vi "On Drop.vi"(8 "error in (no error)":errorcluster, 10 "Actor in":refnum<class "Actor.lvclass">, 11 "Client Connection Handler Msg in":refnum<class "Client Connection Handler Msg.lvclass">) -> (0 "error out":errorcluster, 2 "Actor out":refnum<class "Actor.lvclass">, 3 "Client Connection Handler Msg out":refnum<class "Client Connection Handler Msg.lvclass">)   [LabVIEW 2021, in "Echo Broadcast With Server Manager.lvlib" / "Client Connection Handler Msg.lvclass"]
uses:
  Client Connection Handler Msg.lvclass
  <vilib>/ActorFramework/Actor/Actor.lvclass
  WS Client Subscriber/WS Client Subscriber.lvclass
  C:/Program Files/National Instruments/LabVIEW 2021/vi.lib/ActorFramework/Actor/Actor.lvclass
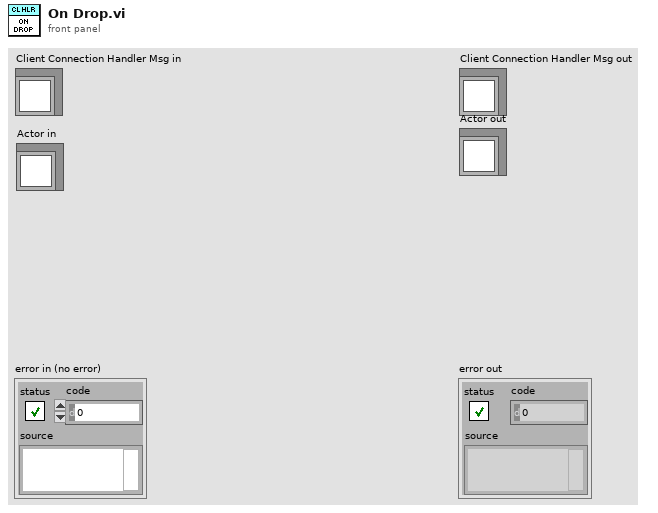
[diagram p1: front panel]
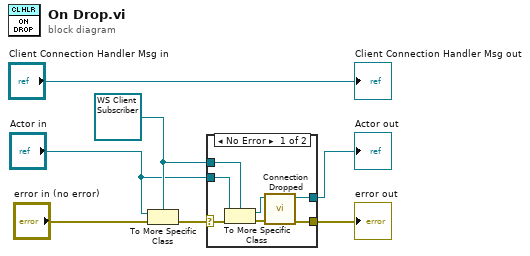
[diagram p0: block diagram]
diagram:
  w3 = refnum<class "WS Client Subscriber.lvclass"> refnum ("WS Full LabVIEW Test.lvlib:WS Test Client.lvclass")
  n1 = To More Specific Class(target class=w3, reference="Actor in", error in="error in (no error)") -> (error out=w5:errorcluster)  [unwired: 1 out]
  n2 = case shown="No Error" w5 {
    selector: w5 -> [w13 w15]
    tunnel: [w14 w15] -> w4
    tunnel: w3 -> [w11 w16]
    tunnel: "Actor in" -> [w10 _]
    tunnel: [w8 w16] -> w1
    frame No Error {
      n3 = To More Specific Class(target class=w11, reference=w10, error in=w13) -> (specific class reference=w9:refnum<class "WS Client Subscriber.lvclass">, error out=w12:errorcluster)
      n4 = call "Connection Dropped.vi"("error in (no error)"=w12, "WS Test Client Subscriber in"=w9) -> ("error out"=w14:errorcluster, "WS Test Client Subscriber out"=w8:refnum<class "WS Client Subscriber.lvclass">)  [unwired: 8 in]
    }
    frame Error {
    }
  }
  "error out" <- w4
  "Actor out" <- w1
  "Client Connection Handler Msg out" <- "Client Connection Handler Msg in"
